vi "TCP-IP Q_Bridge.Create.vi"(4 "Auto Exit":bool, 5 "Notification":bool, 6 "Config":T1={"IP"="127.0.0.1", "Port"=8500, "Listener"=FALSE, "Enable"=FALSE}, 7 "StatusCtrlRef":refnum<vi>, 8 "error in (no error)":errorcluster, 9 "Q_DataOut":refnum<queue> caption="Q_DataOut(To TCP-IP)", 10 "Q_DataIn":refnum<queue> caption="Q_DataIn(From TCP-IP)", 11 "Control Q Name":string="TCP-IP_Bridge") -> (0 "Error Out":errorcluster, 3 "Control Q Dup":string)   [LabVIEW 2024, in "EQMF.lvlib" / "TCP-IP.lvlib"]
uses:
  TCP-IP.lvlib
  Queues/Q.Element.ctl
  Mgr/TCP-IP Mgr.Config.ctl
  _Core/TCP-IP Q_Bridge.Core.vi
  Queues/Queue Utils.lvlib
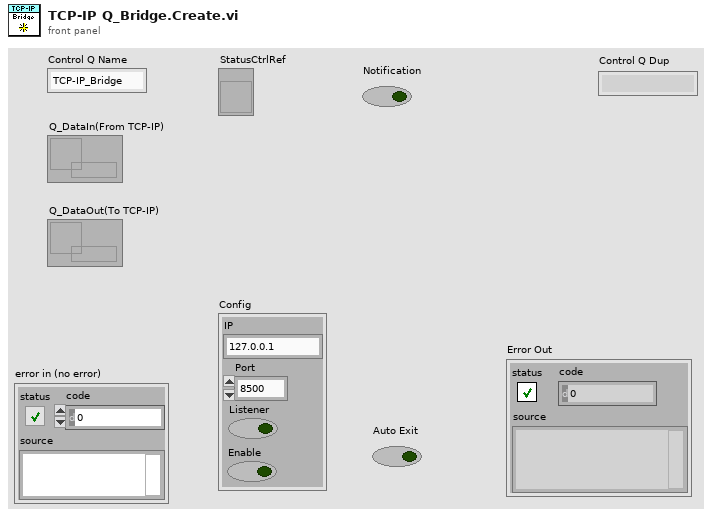
[diagram p1: front panel]
types:
  T1 = typedef "EQMF.lvlib/TCP-IP.lvlib/TCP-IP Mgr.Config.ctl" = cluster{"IP":string, "Port":u16, "Listener":bool, "Enable":bool}
  T2 = cluster{"Controls":cluster{"Ctrl Name":string, "Value":variant}[], "VI Ref":refnum<vi>}
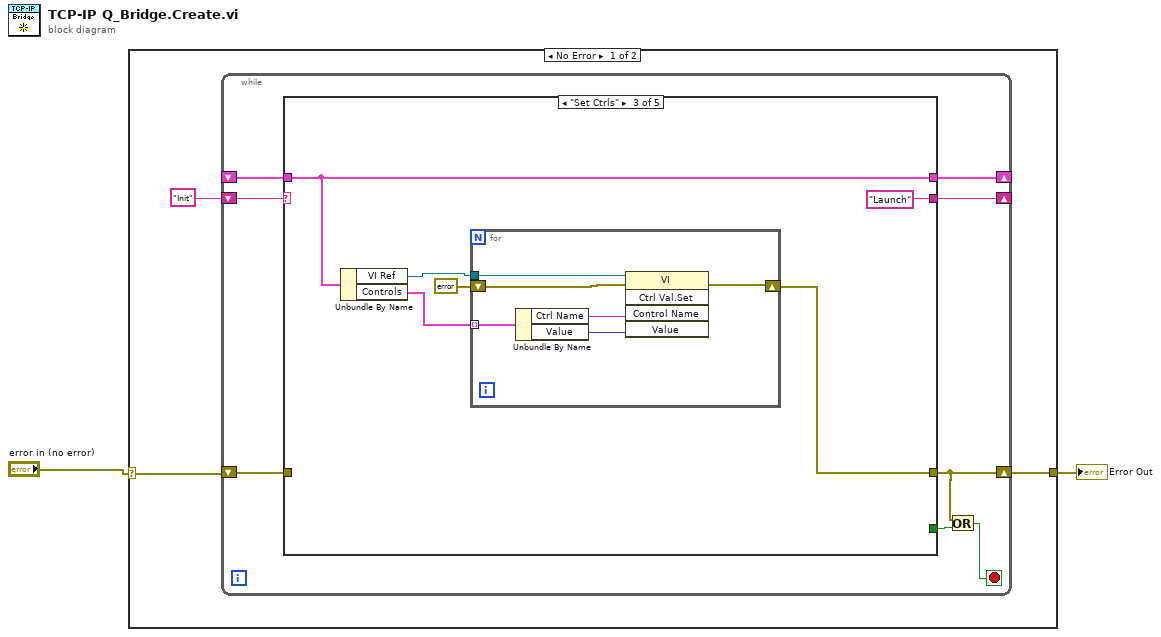
[diagram p0: block diagram]
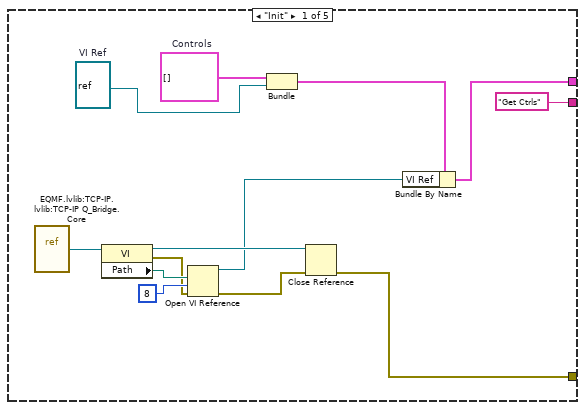
[diagram p2: hidden frame]
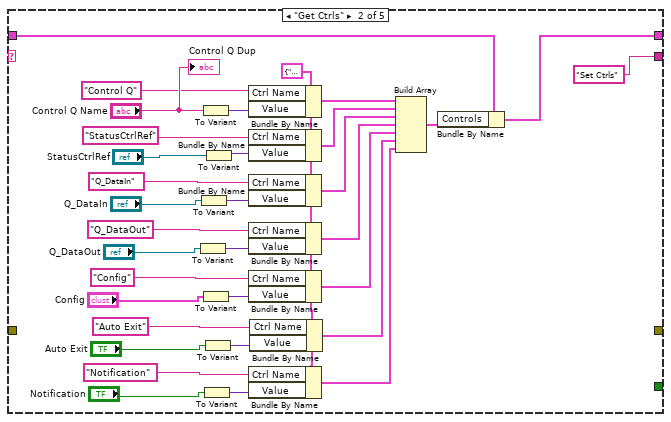
[diagram p3: hidden frame]
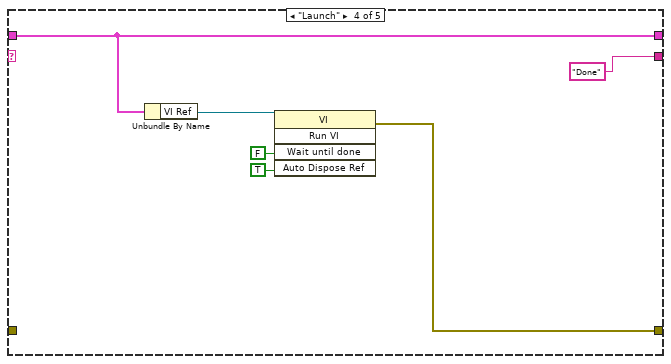
[diagram p4: hidden frame]
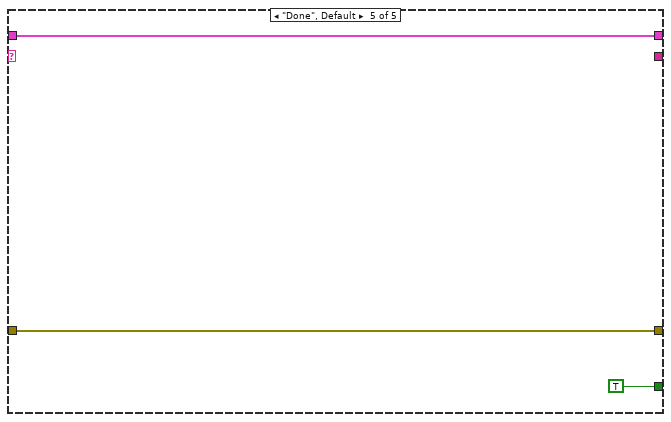
[diagram p5: hidden frame]
diagram:
  n1 = case shown="No Error" "error in (no error)" {
    selector: "error in (no error)" -> [w3 w81]
    tunnel: [w4 w81] -> w2
    frame No Error {
      n2 = while {
        shift-right: [w12] -> _
        shift-left: "Init" -> [w13]
        shift-right: [w10] -> _
        shift-left: _ -> [w11]
        shift-right: [w7] -> w4
        shift-left: w3 -> [w9]
        stop <- w6 stop-if-true
        n3 = case shown="\"Set Ctrls\"" w13 {
          tunnel: [_ _ _ _ TRUE] -> w8
          tunnel: ["Get Ctrls" "Set Ctrls" "Launch" "Done" _] -> w12
          tunnel: w11 -> [_ w35 w64 w74 w79]
          tunnel: [w23 w34 w64 w74 w79] -> w10
          tunnel: w9 -> [_ _ _ _ w78]
          tunnel: [w14 _ w60 w72 w78] -> w7
          frame "Init" {
            w16 = refnum<vi> refnum  # VI Ref
            w25 = cluster{"Ctrl Name":string, "Value":variant}[] []  # Controls
            n4 = vi-ref "EQMF.lvlib:TCP-IP.lvlib:TCP-IP Q_Bridge.Core.vi"() -> (w22:refnum<vi>)
            n5 = property class="VI"(reference=w22) -> (reference out=w20:refnum<vi>, error out=w17:errorcluster, "Path"=w21:path)  [unwired: 1 in]
            n6 = Open VI Reference(vi path=w21, options=8, error in (no error)=w17) -> (vi reference=w15:refnum<vi>, error out=w19:errorcluster)  [unwired: 3 in]
            n7 = Bundle("Controls"=w25, "VI Ref"=w16) -> (w24:T2)  [unwired: 1 in]
            n8 = Close Reference(reference=w20, error in (no error)=w19) -> (error out=w14:errorcluster)
            n9 = Bundle By Name(cluster=w24, "VI Ref"=w15) -> (w23:T2)
          }
          frame "Get Ctrls" {
            w29 = cluster{"Ctrl Name":string, "Value":variant} {"Ctrl Name"="", "Value"=variant} ("Cluster")
            n10 = To Variant(anything="Q_DataOut") -> (Variant=w49:variant)
            n11 = To Variant(anything="Q_DataIn") -> (Variant=w55:variant)
            n12 = To Variant(anything="Control Q Name") -> (Variant=w54:variant)
            n13 = To Variant(anything="Config") -> (Variant=w46:variant)
            n14 = To Variant(anything="Notification") -> (Variant=w30:variant)
            n15 = To Variant(anything="Auto Exit") -> (Variant=w45:variant)
            n16 = To Variant(anything="StatusCtrlRef") -> (Variant=w53:variant)
            n17 = Bundle By Name(cluster=w29, "Ctrl Name"="Control Q", "Value"=w54) -> (w57:cluster{"Ctrl Name":string, "Value":variant})
            n18 = Bundle By Name(cluster=w29, "Ctrl Name"="StatusCtrlRef", "Value"=w53) -> (w58:cluster{"Ctrl Name":string, "Value":variant})
            n19 = Bundle By Name(cluster=w29, "Ctrl Name"="Q_DataIn", "Value"=w55) -> (w56:cluster{"Ctrl Name":string, "Value":variant})
            n20 = Bundle By Name(cluster=w29, "Ctrl Name"="Q_DataOut", "Value"=w49) -> (w47:cluster{"Ctrl Name":string, "Value":variant})
            n21 = Bundle By Name(cluster=w29, "Ctrl Name"="Config", "Value"=w46) -> (w42:cluster{"Ctrl Name":string, "Value":variant})
            n22 = Bundle By Name(cluster=w29, "Ctrl Name"="Notification", "Value"=w30) -> (w28:cluster{"Ctrl Name":string, "Value":variant})
            n23 = Bundle By Name(cluster=w29, "Ctrl Name"="Auto Exit", "Value"=w45) -> (w41:cluster{"Ctrl Name":string, "Value":variant})
            n24 = Build Array(w57, w58, w56, w47, w42, w41, w28) -> (w33:cluster{"Ctrl Name":string, "Value":variant}[])
            n25 = Bundle By Name(cluster=w35, "Controls"=w33) -> (w34:T2)
            "Control Q Dup" <- "Control Q Name"
          }
          frame "Set Ctrls" {
            n26 = Unbundle By Name(w64) -> ("VI Ref"=w63:refnum<vi>, "Controls"=w61:cluster{"Ctrl Name":string, "Value":variant}[])
            n27 = for {
              shift-right: [w69] -> w60
              shift-left: errorcluster {"status"=FALSE, "code"=0, "source"=""} ("error out") -> [w70]
              tunnel: w61 -> [w68] mode=indexing
              tunnel: w63 -> [w71]
              n28 = Unbundle By Name(w68) -> ("Ctrl Name"=w66:string, "Value"=w67:variant)
              n29 = invoke class="VI" method="Ctrl Val.Set"(reference=w71, error in=w70, "Control Name"=w66, "Value"=w67) -> (error out=w69:errorcluster)  [unwired: 1 in, 4 out]
            }
          }
          frame "Launch" {
            n30 = Unbundle By Name(w74) -> ("VI Ref"=w73:refnum<vi>)
            n31 = invoke class="VI" method="Run VI"(reference=w73, "Wait until done"=FALSE ("Wait Until Done"), "Auto Dispose Ref"=TRUE ("Auto Dispose Reference")) -> (error out=w72:errorcluster)  [unwired: 2 in, 4 out]
          }
          frame "Done", Default {
          }
        }
        n32 = Or(x=w7, y=w8) -> (x .or. y?=w6:bool)
      }
    }
    frame Error {
    }
  }
  "Error Out" <- w2
